vi "getType(rec).vi"(6 "clusterIndex (stop) 2":i32[](array[numeric]), 7 "index":i32, 9 "clusterIndex (start)":i32[](array[numeric]), 10 "variant in":variant, 11 "type in":T1[](array[typedef]) format="%.0x") -> (0 "clusterIndex (start)":i32[](array[numeric]), 1 "Cluster Names":string[](array[string]), 2 "Array 2":variant[](array[variant]), 3 "Array":T1[](array[typedef]) format="%.0x", 4 "clusterIndex (stop)":i32[](array[numeric]), 5 "index 2":i32)   [LabVIEW 2011]
uses:
  <userlib>/_OpenG.lib/lvdata/lvdata.llb/Type Descriptor Enumeration__ogtk.ctl
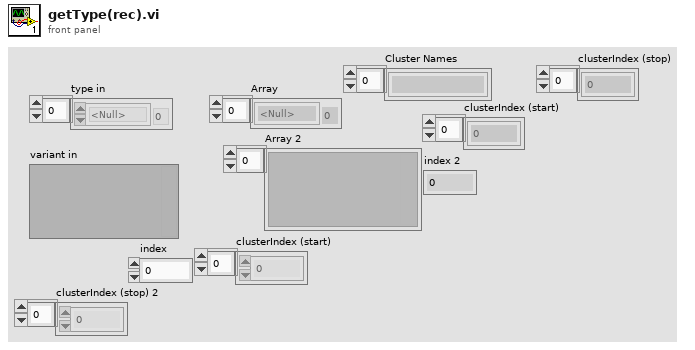
[diagram p1: front panel]
types:
  T1 = typedef "Type Descriptor Enumeration__ogtk.ctl" = enum8{"<Null>", "I8", "I16", "I32", "I64", "U8", "U16", "U32", "U64", "SGL", "DBL", "EXT", "CSG", "CDB", "CXT", "0x0F", "0x10", "0x11", "0x12", "0x13", "0x14", "Enum U8", "Enum U16", "Enum U32", "Enum U64", "SGL PQ", "DBL PQ", "EXT PQ", "CSG PQ", "CDB PQ", "CXT PQ", "0x1F", "0x20", "Boolean", "0x22", "0x23", "0x24", "0x25", "0x26", "0x27", "0x28", "0x29", "0x2A", "0x2B", "0x2C", "0x2D", "0x2E", "0x2F", "String", "0x31", "Path", "Pict", "0x34", "0x35", "0x36", "DAQ", "0x38", "0x39", "0x3A", "0x3B", "0x3C", "0x3D", "0x3E", "0x3F", "Array", "0x41", "0x42", "0x43", "0x44", "0x45", "0x46", "0x47", "0x48", "0x49", "0x4A", "0x4B", "0x4C", "0x4D", "0x4E", "0x4F", "Cluster", "0x51", "0x52", "Variant", "Waveform", "0x55", "0x56", "0x57", "0x58", "0x59", "0x5A", "0x5B", "0x5C", "0x5D", "0x5E", "0x5F", "0x60", "0x61", "0x62", "0x63", "0x64", "0x65", "0x66", "0x67", "0x68", "0x69", "0x6A", "0x6B", "0x6C", "0x6D", "0x6E", "0x6F", "Refnum"}
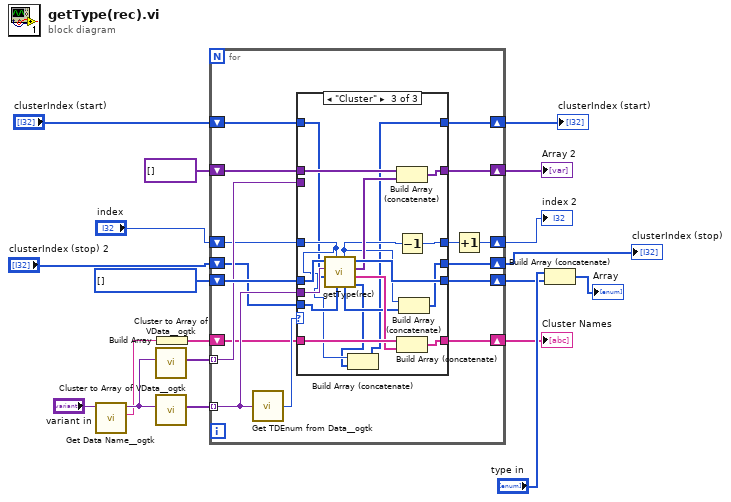
[diagram p0: block diagram]
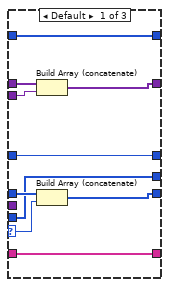
[diagram p2: hidden frame]
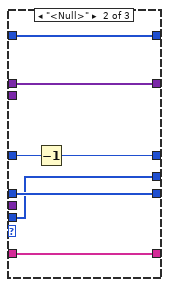
[diagram p3: hidden frame]
diagram:
  w15 = T1[] [] items=["<Null>", "I8", "I16", "I32", "I64", "U8", "U16", "U32", "U64", "SGL", "DBL", "EXT", "CSG", "CDB", "CXT", "0x0F", "0x10", "0x11", "0x12", "0x13", "0x14", "Enum U8", "Enum U16", "Enum U32", "Enum U64", "SGL PQ", "DBL PQ", "EXT PQ", "CSG PQ", "CDB PQ", "CXT PQ", "0x1F", "0x20", "Boolean", "0x22", "0x23", "0x24", "0x25", "0x26", "0x27", "0x28", "0x29", "0x2A", "0x2B", "0x2C", "0x2D", "0x2E", "0x2F", "String", "0x31", "Path", "Pict", "0x34", "0x35", "0x36", "DAQ", "0x38", "0x39", "0x3A", "0x3B", "0x3C", "0x3D", "0x3E", "0x3F", "Array", "0x41", "0x42", "0x43", "0x44", "0x45", "0x46", "0x47", "0x48", "0x49", "0x4A", "0x4B", "0x4C", "0x4D", "0x4E", "0x4F", "Cluster", "0x51", "0x52", "Variant", "Waveform", "0x55", "0x56", "0x57", "0x58", "0x59", "0x5A", "0x5B", "0x5C", "0x5D", "0x5E", "0x5F", "0x60", "0x61", "0x62", "0x63", "0x64", "0x65", "0x66", "0x67", "0x68", "0x69", "0x6A", "0x6B", "0x6C", "0x6D", "0x6E", "0x6F", "Refnum"]
  n1 = call <userlib>:"Get Data Name__ogtk.vi"("Data"="variant in") -> ("Data Name"=w9:string, "Data dup"=w10:variant)  [unwired: 8 in, 1 out]
  n2 = call <userlib>:"Cluster to Array of VData__ogtk.vi"("Cluster"=w10) -> ("Array of VData"=w14:variant[])  [unwired: 9 in, 1 out]
  n3 = call <userlib>:"Cluster to Array of VData__ogtk.vi"("Cluster"=w10) -> ("Array of VData"=w17:variant[])  [unwired: 9 in, 1 out]
  n4 = Build Array(w9) -> (w8:string[])
  n5 = for {
    tunnel: w17 -> [w35] mode=indexing
    shift-right: [w33] -> w16
    shift-left: w15 -> [w34]
    tunnel: w14 -> [w31] mode=indexing
    shift-right: [w30] -> w13
    shift-left: variant[] [] -> [w29]
    shift-right: [w27] -> w7
    shift-left: w8 -> [w28]
    shift-right: [w25] -> w4
    shift-left: "clusterIndex (start)" -> [w26]
    shift-right: [w23] -> w5
    shift-left: "index" -> [w22]
    shift-right: [w21] -> w2
    shift-left: "clusterIndex (stop) 2" -> [w20]
    n6 = call <userlib>:"Get TDEnum from Data__ogtk.vi"("Data"=w35) -> ("Type Descriptor Enumeration"=w32:T1)  [unwired: 4 in]
    n7 = case shown="\"Cluster\"" w32 {
      selector: w32 -> [w45 _ _]
      tunnel: w35 -> [_ _ w70]
      tunnel: w34 -> [w44 w52 w69]
      tunnel: [w43 w52 w68] -> w33
      tunnel: w31 -> [w42 _ _]
      tunnel: [w41 w51 w65] -> w30
      tunnel: w29 -> [w40 w51 w66]
      tunnel: w28 -> [w39 w50 w64]
      tunnel: [w39 w50 w62] -> w27
      tunnel: w26 -> [w38 w49 w55]
      tunnel: [w38 w49 w53] -> w25
      tunnel: w22 -> [w37 w47 w56]
      tunnel: [w37 w46 w61] -> w24
      tunnel: [w36 w48 w60] -> w21
      tunnel: w20 -> [w36 w48 w59]
      frame Default {
        n8 = Build Array (concatenate)(w40, w42) -> (w41:variant[])
        n9 = Build Array (concatenate)(w44, w45) -> (w43:T1[])
      }
      frame "<Null>" {
        n10 = Decrement(x=w47) -> (x-1=w46:i32)
      }
      frame "Cluster" {
        n11 = call "getType(rec).vi"("clusterIndex (stop) 2"=w59, "index"=w56, "clusterIndex (start)"=w55, "variant in"=w70, "type in"=w69) -> ("clusterIndex (start)"=w54:i32[], "Cluster Names"=w63:string[], "Array 2"=w67:variant[], "Array"=w68:T1[], "clusterIndex (stop)"=w58:i32[], "index 2"=w57:i32)  [unwired: 1 in]
        n12 = Build Array (concatenate)(w56, w54) -> (w53:i32[])
        n13 = Build Array (concatenate)(w66, w67) -> (w65:variant[])
        n14 = Decrement(x=w57) -> (x-1=w61:i32)
        n15 = Build Array (concatenate)(w64, w63) -> (w62:string[])
        n16 = Build Array (concatenate)(w57, w58) -> (w60:i32[])
      }
    }
    n17 = Increment(x=w24) -> (x+1=w23:i32)
  }
  "Array 2" <- w13
  "Cluster Names" <- w7
  "clusterIndex (start)" <- w4
  "index 2" <- w5
  "clusterIndex (stop)" <- w2
  n18 = Build Array (concatenate)("type in", w16) -> (→"Array":T1[])
